vi "Window Calc.vi"() -> ()   [LabVIEW 2013]
uses:
  <vilib>/Analysis/4window.llb/Hanning Window (DBL).vi
  <vilib>/Analysis/4window.llb/AllCosWindow (DBL).vi
  <vilib>/Analysis/NI_AALPro.lvlib
panel:
  out "sum":dbl
  out "Waveform Graph 2":dbl[](graph)
  out "max index(es)":i32
  out "max value":dbl
  out "Waveform Graph":dbl[](graph)
  out "Windowed X":dbl[](array[numeric])
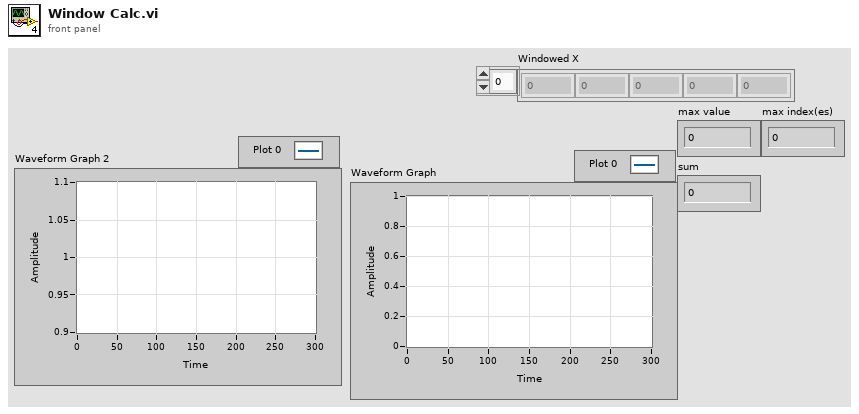
[diagram p1: front panel]
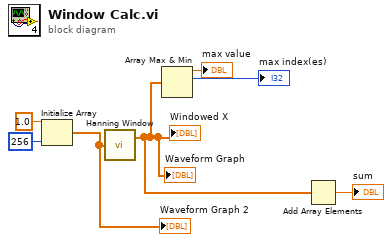
[diagram p0: block diagram]
diagram:
  n1 = Initialize Array(1.0 ("element"), 256 ("dimension size")) -> (w3:dbl[])
  "Waveform Graph 2" <- w3
  n2 = call-poly <vilib>:"Hanning Window.vi"("X"=w3) -> ("Windowed X"=w2:dbl[])  [unwired: 1 out]
  "Windowed X" <- w2
  "Waveform Graph" <- w2
  n3 = Array Max & Min(array=w2) -> (max value=→"max value":dbl, max index (indices)=→"max index(es)":i32)  [unwired: 2 out]
  n4 = Add Array Elements(numeric array=w2) -> (sum=→"sum":dbl)
